vi "RSZVB Save Pulse Train File.vi"(7 "File Name (\"\")":string, 8 "error in (no error)":errorcluster {"code" format="%.0x"}, 9 "Generator (1)":i32=1, 10 "Channel (1)":i32=1, 11 "VISA session":refnum<visa-resource-name>) -> (0 "error out":errorcluster {"code" format="%.0x"}, 3 "dup VISA session":refnum<visa-resource-name>)   [LabVIEW 2011]
doc: "This VI saves a pulse train definition associated with a specified channel to a pulse train file.\n\nNote(s):\n\n(1) This VI is available only with option R&S ZVA-K27.\n\nRemote-control command(s):\nMMEMory:STORe:PTRain <Channel>, <Generator>, '<file_name>'"
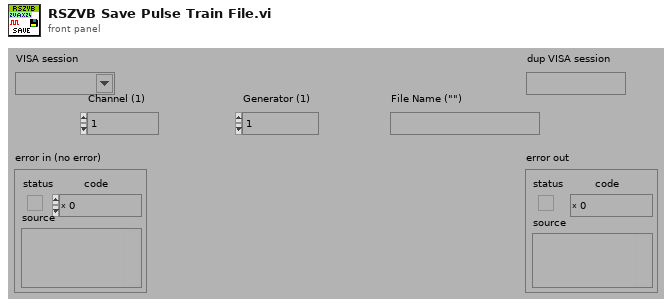
[diagram p1: front panel]
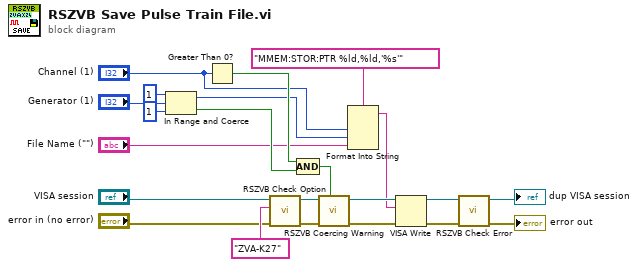
[diagram p0: block diagram]
diagram:
  n1 = In Range and Coerce(upper limit=1, x="Generator (1)", lower limit=1) -> (coerced(x)=w3:i32, In Range?=w5:bool)
  n2 = Greater Than 0?(x="Channel (1)") -> (x > 0?=w12:bool)
  n3 = call "RSZVB Check Option.vi"("error in (no error)"="error in (no error)", "Options"="ZVA-K27", "VISA session"="VISA session") -> ("error out"=w16:errorcluster, "dup VISA session"=w15:refnum<visa-resource-name>)  [unwired: 7 in]
  n4 = Compound Arithmetic op=AND(w12, w5) -> (w14:bool)
  n5 = call "RSZVB Coercing Warning.vi"("In Range?"=w14, "error in (no error)"=w16, "VISA session"=w15) -> ("error out"=w21:errorcluster, "dup VISA session"=w22:refnum<visa-resource-name>)  [unwired: 7 in]
  n6 = Format Into String(format string="MMEM:STOR:PTR %ld,%ld,'%s'", "Channel (1)", w3, "File Name (\"\")") -> (resulting string=w18:string)  [unwired: 2 in, 1 out]
  n7 = VISA Write(VISA resource name=w22, write buffer=w18, error in (no error)=w21) -> (VISA resource name out=w19:refnum<visa-resource-name>, error out=w20:errorcluster)  [unwired: 1 out]
  n8 = call "RSZVB Check Error.vi"("error in (no error)"=w20, "VISA session"=w19) -> ("error out"=→"error out":errorcluster, "dup VISA session"=→"dup VISA session":refnum<visa-resource-name>)  [unwired: 8 in]
